vi "Msg - Receive Module Data.vi"(11 "error in (no error)":errorcluster) -> (4 "Module Data Out":T1, 15 "error out":errorcluster)   [LabVIEW 2016, in "Template.lvlib"]
doc: "Allows controller to receive the Module Data of THIS Module"
uses:
  Template.lvlib
  Controls/Module - Data.ctl
  Modules.ctl
  Controls/Module - States.ctl
  Controls/Timing - Data.ctl
  Controls/Process - Element.ctl
  Controls/Process.ctl
  Controls/Process - Status.ctl
  Controls/Message - Queue Manager Mode.ctl
  Controls/Message.ctl
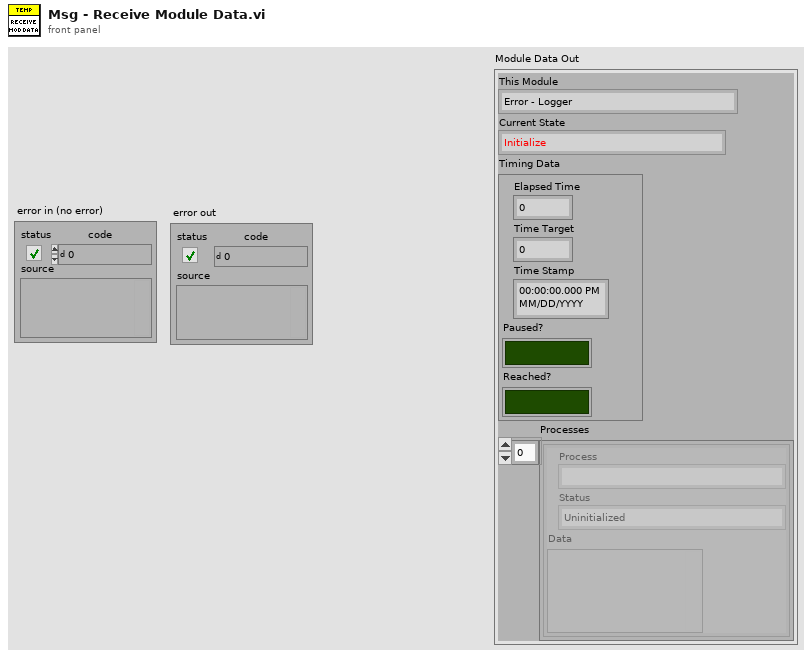
[diagram p1: front panel]
types:
  T1 = typedef "Template.lvlib/Module - Data.ctl" = cluster{"This Module":T2, "Current State":T3, "Timing Data":T4, "Processes":T5[]}
  T2 = typedef "Modules.ctl" = enum16{"Error - Logger", "Hardware Interface", "UI Handler", "Database Handler"}
  T3 = typedef "Template.lvlib/Module - States.ctl" = enum16{"Initialize", "Event ", "Send data", "FP Element: Update", "FP Element: Disable/Enable", "Timer: Setup", "Terminate", "---------------Template---------------"}
  T4 = typedef "Template.lvlib/Timing - Data.ctl" = cluster{"Elapsed Time":dbl, "Time Target":dbl, "Time Stamp":timestamp, "Paused?":bool, "Reached?":bool}
  T5 = typedef "Template.lvlib/Process - Element.ctl" = cluster{"Process":T6, "Status":T7, "Data":variant}
  T6 = typedef "Template.lvlib/Process.ctl" = enum16{""}
  T7 = typedef "Template.lvlib/Process - Status.ctl" = enum16{"Uninitialized", "Busy"}
  T8 = typedef "Template.lvlib/Message.ctl" = cluster{"State":T3, "Data":variant, "Transitioning State?":bool}
  T9 = typedef "Template.lvlib/Message - Queue Manager Mode.ctl" = enum16{"Create", "Get", "Destroy"}
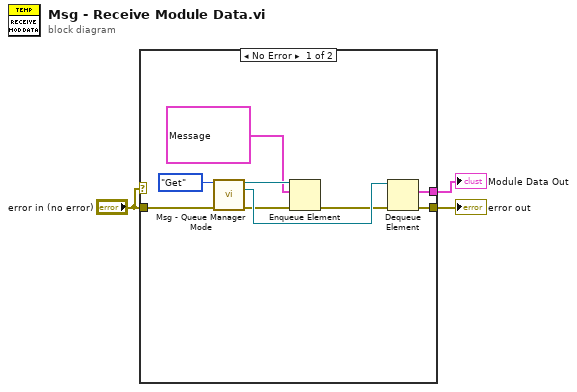
[diagram p0: block diagram]
diagram:
  n1 = case shown="No Error" "error in (no error)" {
    tunnel: [w9 _] -> w3
    tunnel: [w7 w12] -> w2
    tunnel: "error in (no error)" -> [w8 w12]
    frame No Error {
      n2 = call "Msg - Queue Manager Mode.vi"("Mode"=Message_-_Queue_Manager_Mode."Get", "error in (no error)"=w8) -> (">>ThisModule"=w5:refnum<queue>, ">>Controller"=w10:refnum<queue>, "error out"=w6:errorcluster)  [unwired: 11 in]
      n3 = Enqueue Element(queue=w5, element=T8 {"State"=enum."Send data", "Data"=variant, "Transitioning State?"=FALSE}, error in (no error)=w6) -> ()  [unwired: 1 in, 3 out]
      n4 = Dequeue Element(queue=w10, error in (no error)=w6) -> (element=w9:T1, error out=w7:errorcluster)  [unwired: 1 in, 2 out]
    }
    frame Error {
    }
  }
  "error out" <- w2
  "Module Data Out" <- w3
